vi "RemoveTermChar.vi"(4 "String":string) -> (1 "Chopped String":string)   [LabVIEW 2024]
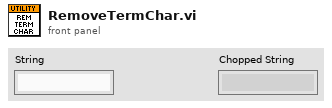
[diagram p1: front panel]
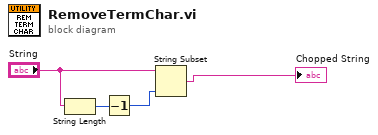
[diagram p0: block diagram]
diagram:
  n1 = String Length(string="String") -> (length=w4:i32)
  n2 = Decrement(x=w4) -> (x-1=w3:i32)
  n3 = String Subset(string="String", length (rest)=w3) -> (substring=→"Chopped String":string)  [unwired: 1 in]
